vi "Reparent Included PPLs.vi"(8 "error in":errorcluster, 11 "custom device project":path) -> (0 "error out":errorcluster)   [LabVIEW 2020, in "Template Tool.lvlib"]
uses:
  Template Tool.lvlib
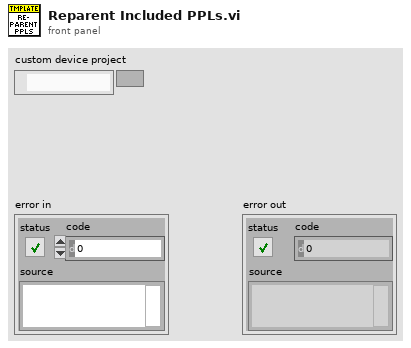
[diagram p1: front panel]
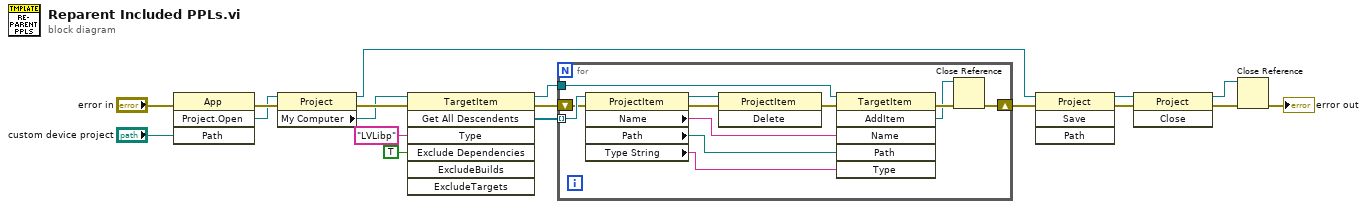
[diagram p0: block diagram]
diagram:
  n1 = invoke class="App" method="Project.Open"(error in="error in", "Path"="custom device project") -> (error out=w18:errorcluster, "Project:Open"=w17:refnum<vi>)  [unwired: 2 in, 2 out]
  n2 = property class="Project"(reference=w17, error in=w18) -> (reference out=w10:refnum<vi>, error out=w16:errorcluster, "My Computer"=w15:refnum<vi>)
  n3 = invoke class="TargetItem" method="Get All Descendents"(reference=w15, error in=w16, "Type"="LVLibp", "Exclude Dependencies"=TRUE ("ExcludeDependencies")) -> (reference out=w11:refnum<vi>, error out=w9:errorcluster, "All Descendents"=w12:refnum<vi>[])  [unwired: 3 in, 4 out]
  n4 = for {
    tunnel: w12 -> [w30] mode=indexing
    shift-right: [w20] -> w8
    shift-left: w9 -> [w27]
    tunnel: w11 -> [w25]
    n5 = property class="ProjectItem"(reference=w30, error in=w27) -> (reference out=w29:refnum<vi>, error out=w28:errorcluster, "Name"=w24:string, "Path"=w23:path, "Type String"=w22:string)
    n6 = invoke class="ProjectItem" method="Delete"(reference=w29, error in=w28) -> (error out=w26:errorcluster)  [unwired: 1 in, 2 out]
    n7 = invoke class="TargetItem" method="AddItem"(reference=w25, error in=w26, "Name"=w24, "Path"=w23, "Type"=w22) -> (error out=w21:errorcluster, "AddItem"=w19:refnum<vi>)  [unwired: 1 in, 4 out]
    n8 = Close Reference(reference=w19, error in (no error)=w21) -> (error out=w20:errorcluster)
  }
  n9 = invoke class="Project" method="Save"(reference=w10, error in=w8) -> (reference out=w6:refnum<vi>, error out=w7:errorcluster)  [unwired: 2 in, 2 out]
  n10 = invoke class="Project" method="Close"(reference=w6, error in=w7) -> (reference out=w4:refnum<vi>, error out=w5:errorcluster)  [unwired: 1 in, 1 out]
  n11 = Close Reference(reference=w4, error in (no error)=w5) -> (error out=→"error out":errorcluster)
